vi "Main_SIA.vi"() -> ()   [LabVIEW 2026]
panel:
  in  "Stop":bool
  in  "CALCULEAZA":bool
  out "Risc Hiper":dbl(knob) scale=0.0..1.0
  out "Risc Inima":dbl(knob) scale=0.0..1.0
  out "Risc Diabet":dbl(knob) scale=0.0..1.0
  in  "Sport":dbl(slide) scale=0.0..10.0
  in  "Puls":dbl(slide) scale=40.0..150.0
  in  "Varsta":dbl(slide) scale=20.0..90.0
  in  "BMI":dbl(slide) scale=15.0..45.0
  in  "Colesterol":dbl(slide) scale=100.0..350.0
  in  "Tensiune":dbl(slide) scale=80.0..200.0
  in  "Glucoza":dbl(slide) scale=50.0..250.0
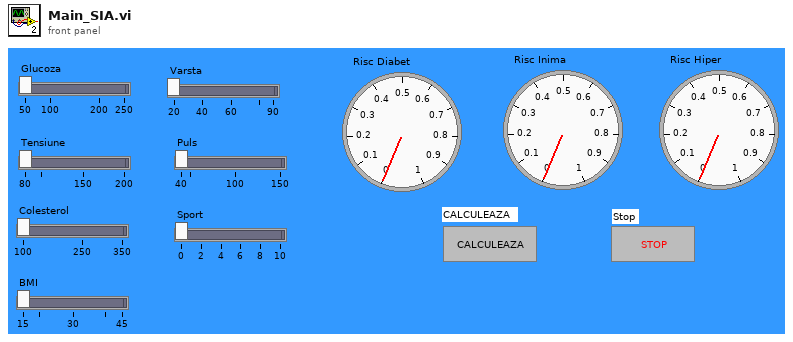
[diagram p1: front panel]
types:
  T1 = enum16{"Idle", "Acquire", "Preprocess", "Inference", "Display"}
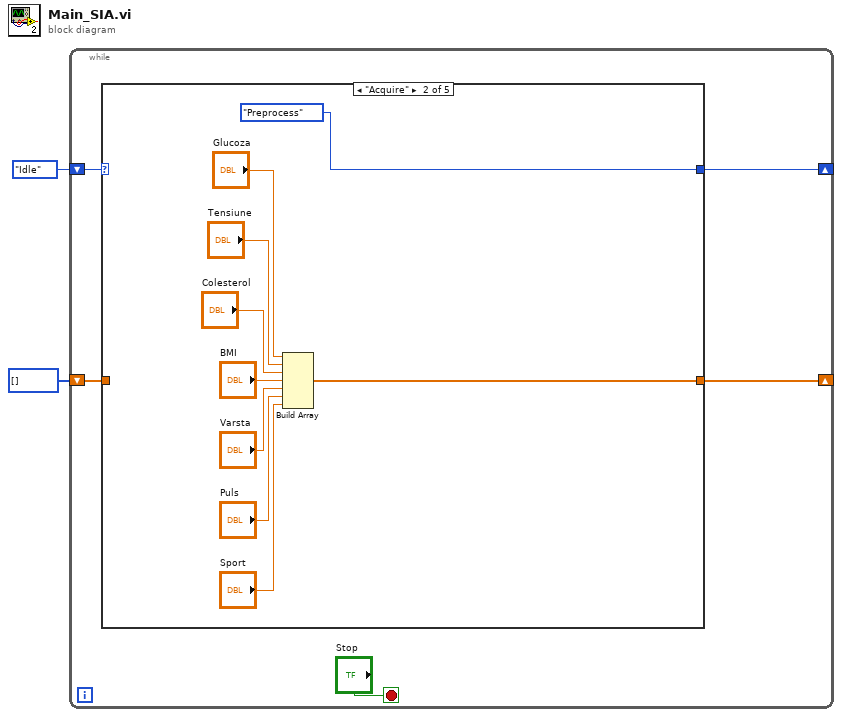
[diagram p0: block diagram]
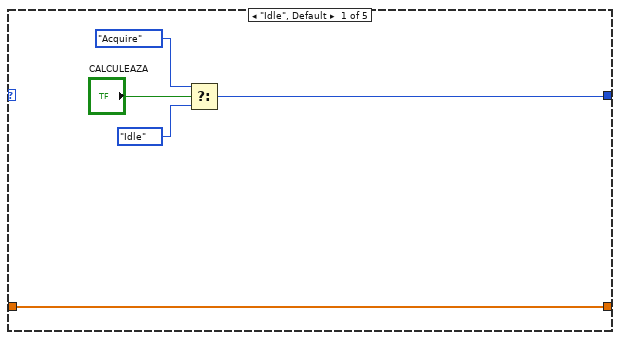
[diagram p2: hidden frame]
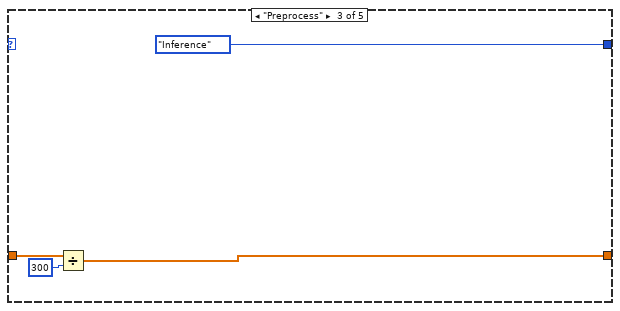
[diagram p3: hidden frame]
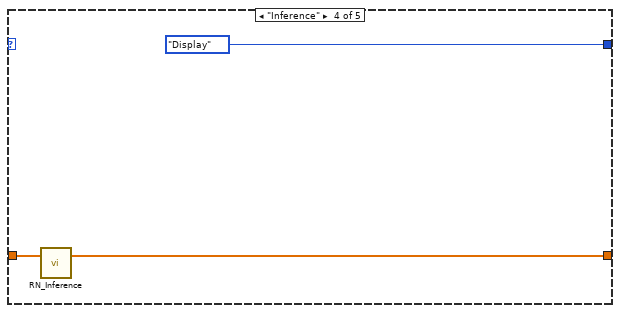
[diagram p4: hidden frame]
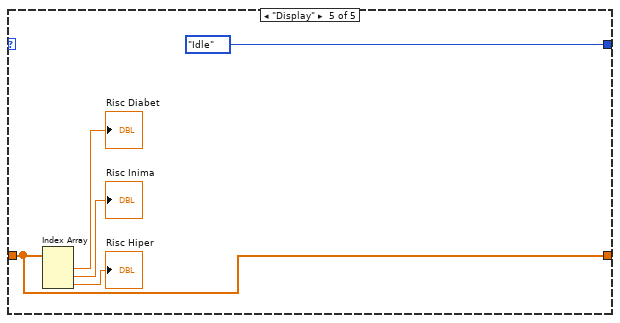
[diagram p5: hidden frame]
diagram:
  n1 = while {
    shift-right: [w6] -> _
    shift-left: T1."Idle" -> [w7]
    shift-right: [w4] -> _
    shift-left: i32[] [] -> [w5]
    stop <- "Stop" stop-if-true
    n2 = case shown="\"Acquire\"" w7 {
      tunnel: [w9 T1."Preprocess" T1."Inference" T1."Display" T1."Idle"] -> w6
      tunnel: w5 -> [w8 _ w25 w28 w29]
      tunnel: [w8 w13 w24 w27 w29] -> w4
      frame "Idle", Default {
        n3 = Select(t=T1."Acquire", s="CALCULEAZA", f=T1."Idle") -> (s? t:f=w9:T1)
      }
      frame "Acquire" {
        n4 = Build Array("Glucoza", "Tensiune", "Colesterol", "BMI", "Varsta", "Puls", "Sport") -> (w13:dbl[])
      }
      frame "Preprocess" {
        n5 = Divide(x=w25, y=300) -> (x/y=w24:dbl[])
      }
      frame "Inference" {
        n6 = call "RN_Inference.vi"("Input Features"=w28) -> ("Output Probabilities"=w27:dbl[])  [unwired: 2 in]
      }
      frame "Display" {
        n7 = Index Array(array=w29) -> (element #1=→"Risc Diabet":dbl, element #2=→"Risc Inima":dbl, element #3=→"Risc Hiper":dbl)  [unwired: 3 in]
      }
    }
  }
